vi "_Read.vi"(8 "error in (no error)":errorcluster, 9 "Timeout S (0)":dbl, 10 "Bytes to Read (0)":i32, 11 "DeployResource in":refnum<class "Resource.lvclass">) -> (0 "error out":errorcluster, 1 "Bytes Read":i32, 2 "Data":string, 3 "DeployResource out":refnum<class "Resource.lvclass">)   [LabVIEW 2020]
uses:
  Resource.lvclass/Resource.ctl
  Resource.lvclass
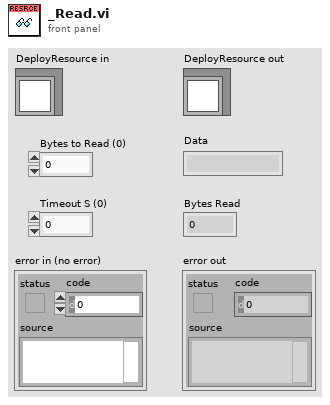
[diagram p1: front panel]
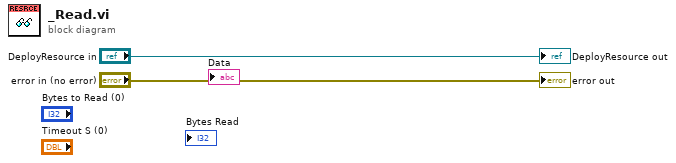
[diagram p0: block diagram]
diagram:
  "error out" <- "error in (no error)"
  "DeployResource out" <- "DeployResource in"
